vi "LogotipoUPIITAFinalV.vi"() -> ()   [LabVIEW 2016]
uses:
  <vilib>/DAQmx/write.llb/DAQmx Write (Analog 2D DBL NChan NSamp).vi
  <vilib>/DAQmx/create/channels.llb/DAQmx Create Channel (AO-Voltage-Basic).vi
  <vilib>/DAQmx/configure/timing.llb/DAQmx Timing (Sample Clock).vi
  <vilib>/DAQmx/miscellaneous.llb/DAQmx Fill In Error Info.vi
panel:
  out "Waveform Graph Y":dbl[](graph)
  out "Waveform Graph X":dbl[](graph)
  out "Tamano_X":i32
  out "XY Graph DAC":cluster{dbl[], dbl[]}(graph)
  out "Columnas":i32
  out "Filas":i32
  out "XY Graph":cluster{i32[], i32[]}(graph)
  out "Array 2":i32[](array[numeric])
  out "Array":i32[](array[numeric])
  out "1-bit pixmap":bool[][](array[boolean])
  out "Logotipo":picture
  in  "File Path":path
  in  "Stop Button":bool
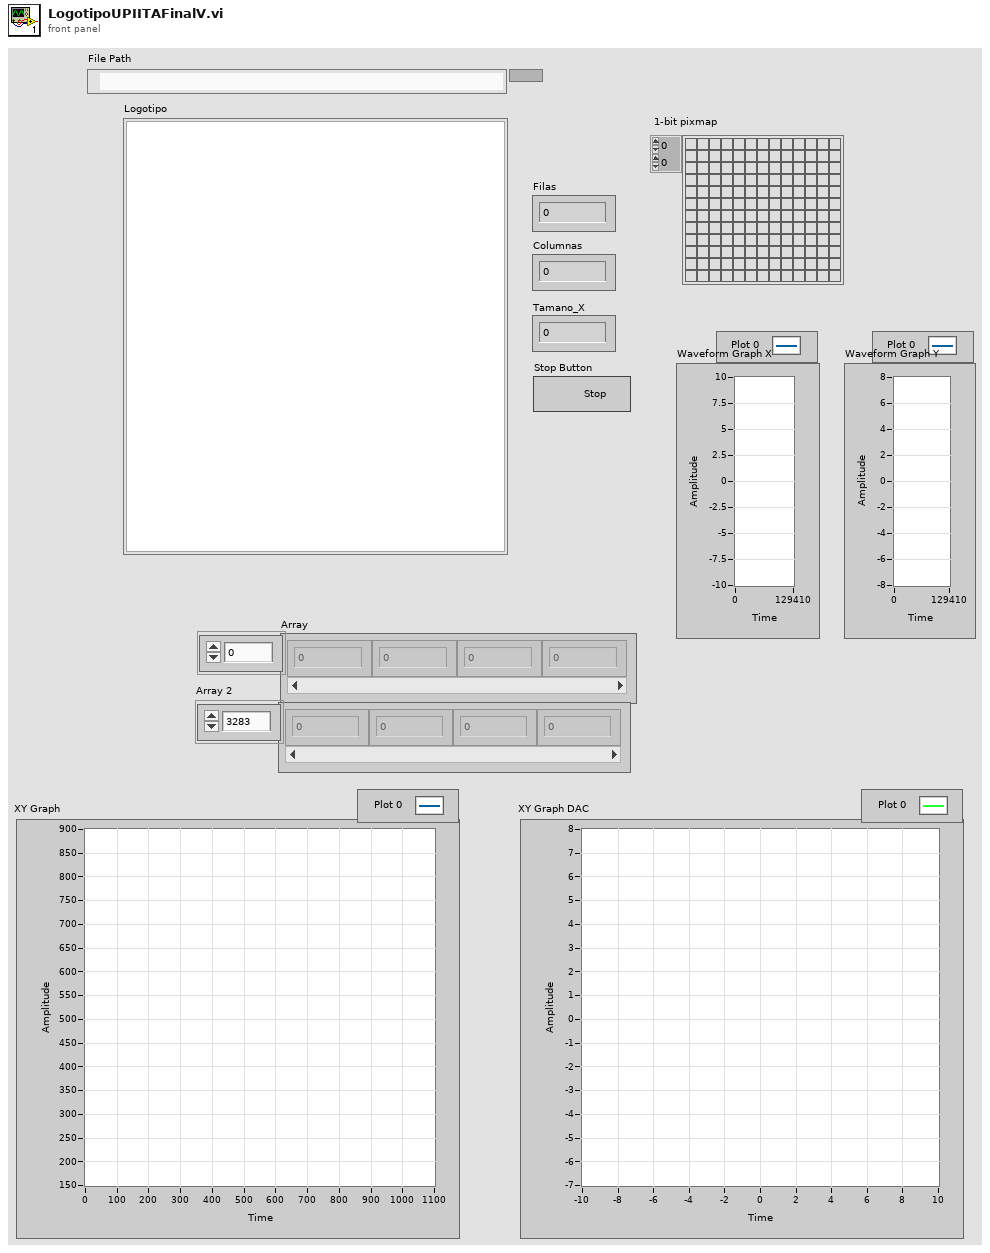
[diagram p1: front panel]
types:
  T1 = typedef "imagedata.ctl" = cluster{"image type":i32, "image depth":i32, "image":u8[], "mask":u8[], "colors":u32[], "Rectangle":cluster{"left":i16, "top":i16, "right":i16, "bottom":i16}}
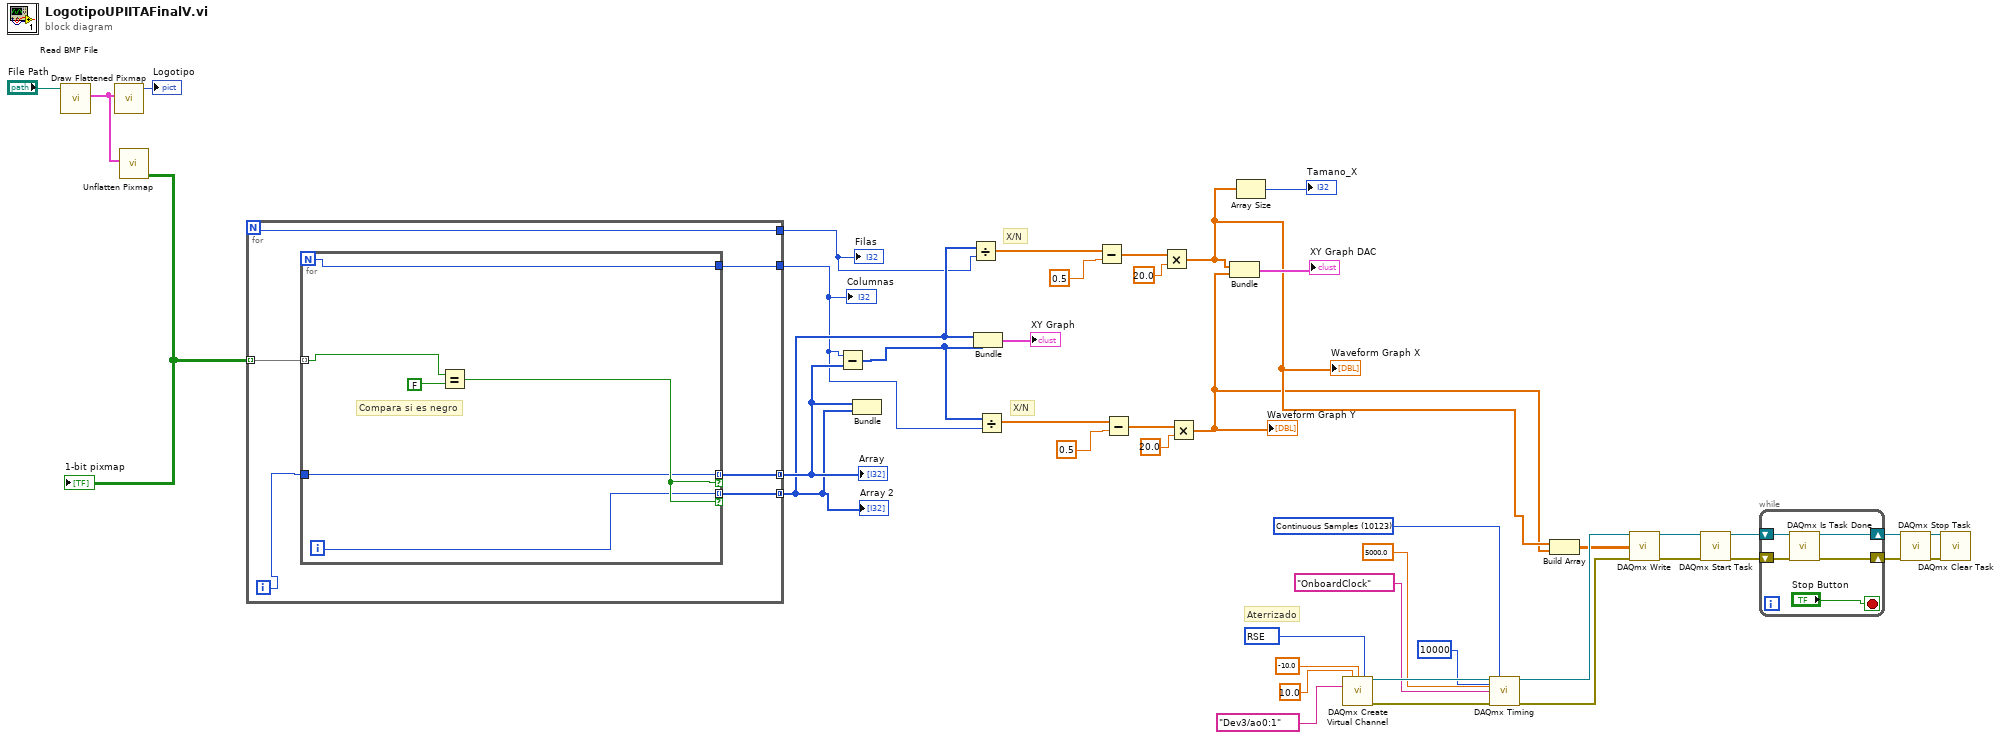
[diagram p0: block diagram]
diagram:
  w3 = 10123 items=["Finite Samples"=10178, "Continuous Samples"=10123, "Hardware Timed Single Point"=12522] ("sample mode")
  w41 = 10083 items=["Default"=-1, "RSE"=10083, "NRSE"=10078, "Differential"=10106, "Pseudodifferential"=12529] ("input terminal configuration")
  # "X/N"
  # "X/N"
  # "Aterrizado"
  n1 = call <vilib>:"Read BMP File.vi"("path to BMP file"="File Path") -> ("image data"=w21:T1)  [unwired: 8 in, 2 out]
  n2 = call <vilib>:"Draw Flattened Pixmap.vi"("image data"=w21) -> ("new picture"=→"Logotipo":picture)  [unwired: 8 in]
  n3 = call <vilib>:"Unflatten Pixmap.vi"("image data"=w21) -> ("1-bit pixmap"=w20:bool[][])  [unwired: 4 in, 6 out]
  "1-bit pixmap" <- w20
  n4 = for {
    N -> [w45]
    tunnel: w20 -> [w49] mode=indexing
    tunnel: [w47] -> w19 mode=concatenating
    tunnel: [w46] -> w17 mode=concatenating
    tunnel: [w45] -> w16
    tunnel: [w44] -> w5
    i -> [w48]
    n5 = for {
      N -> [w50]
      tunnel: w49 -> [w55] mode=indexing
      tunnel: w48 -> [w52]
      tunnel: [w51] -> w46 mode=indexing if=w53
      tunnel: [w52] -> w47 mode=indexing if=w53
      tunnel: [w50] -> w44
      i -> [w51]
      # "Compara si es negro"
      n6 = Equal?(x=w55, y=FALSE) -> (x = y?=w53:bool)
    }
  }
  "Array" <- w19
  "Array 2" <- w17
  "Filas" <- w16
  "Columnas" <- w5
  n7 = Subtract(x=w5, y=w19) -> (x-y=w6:i32[])
  n8 = Bundle(w19, w17) -> ()  [unwired: 1 in, 1 out]
  n9 = Divide(x=w17, y=w16) -> (x/y=w15:dbl[])
  n10 = Bundle(w17, w6) -> (→"XY Graph":cluster{i32[], i32[]})  [unwired: 1 in]
  n11 = Divide(x=w6, y=w5) -> (x/y=w10:dbl[])
  n12 = Subtract(x=w15, y=0.5) -> (x-y=w13:dbl[])
  n13 = Subtract(x=w10, y=0.5) -> (x-y=w8:dbl[])
  n14 = Multiply(x=w13, y=20.0) -> (x*y=w2:dbl[])
  "Waveform Graph X" <- w2
  n15 = Multiply(x=w8, y=20.0) -> (x*y=w1:dbl[])
  "Waveform Graph Y" <- w1
  n16 = Bundle "Bundle"(w2, w1) -> (→"XY Graph DAC":cluster{dbl[], dbl[]})  [unwired: 1 in]
  n17 = Array Size(array=w2) -> (size(s)=→"Tamano_X":i32)
  n18 = call-poly <vilib>:"DAQmx Create Virtual Channel.vi"("maximum value"=10.0, "minimum value"=-10.0, "output terminal configuration"=w41, "physical channels"=tag "Dev3/ao0:1") -> ("task out"=w37:refnum<k21>, "error out"=w36:errorcluster)  [unwired: 10 in]
  n19 = call-poly <vilib>:"DAQmx Timing.vi"("task/channels in"=w37, "sample mode"=w3, "samples per channel"=10000, "rate"=5000.0, "source"=tag "OnboardClock", "error in"=w36) -> ("task out"=w32:refnum<k21>, "error out"=w31:errorcluster)  [unwired: 8 in]
  n20 = Build Array "Build Array"(w2, w1) -> (w24:dbl[][])
  n21 = call-poly <vilib>:"DAQmx Write.vi"("task/channels in"=w32, "data"=w24, "error in"=w31) -> ("task out"=w30:refnum<k21>, "error out"=w29:errorcluster)  [unwired: 10 in, 1 out]
  n22 = call <vilib>:"DAQmx Start Task.vi"("task/channels in"=w30, "error in"=w29) -> ("task out"=w28:refnum<k21>, "error out"=w27:errorcluster)  [unwired: 12 in]
  n23 = while {
    shift-right: [w58] -> w26
    shift-left: w28 -> [w60]
    shift-right: [w57] -> w25
    shift-left: w27 -> [w59]
    stop <- "Stop Button" stop-if-true
    n24 = call <vilib>:"DAQmx Is Task Done.vi"("task/channels in"=w60, "error in"=w59) -> ("task out"=w58:refnum<k21>, "error out"=w57:errorcluster)  [unwired: 11 in, 1 out]
  }
  n25 = call <vilib>:"DAQmx Stop Task.vi"("task/channels in"=w26, "error in"=w25) -> ("task out"=w40:refnum<k21>, "error out"=w39:errorcluster)  [unwired: 12 in]
  n26 = call <vilib>:"DAQmx Clear Task.vi"("task in"=w40, "error in"=w39) -> ()  [unwired: 13 in, 1 out]
